vi "Leer.vi"(0 "VISA resource name out 2":refnum<visa-resource-name>, 1 "error out":errorcluster) -> (2 "Valor":dbl, 3 "VISA resource name out 3":refnum<visa-resource-name>, 4 "error out 2":errorcluster)   [LabVIEW 2015, in "Arduino GIERM.lvlib"]
uses:
  <instrlib>/Arduino GIERM/Arduino GIERM.lvlib
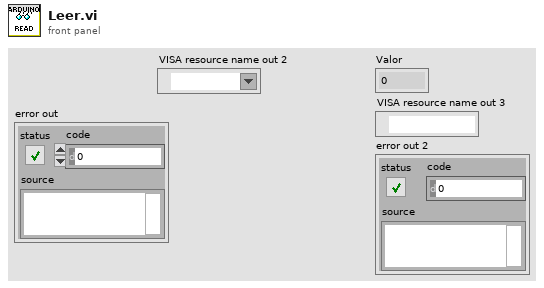
[diagram p1: front panel]
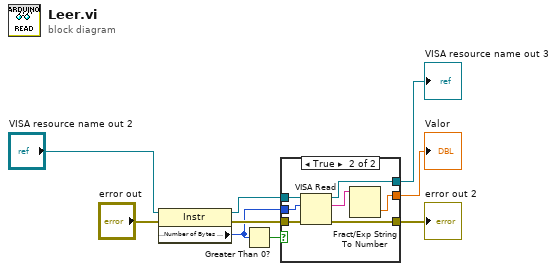
[diagram p0: block diagram]
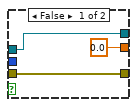
[diagram p2: hidden frame]
diagram:
  n1 = property class="Instr"(reference="VISA resource name out 2", error in="error out") -> (reference out=w5:refnum<visa-resource-name>, error out=w3:errorcluster, "Serial Settings:Number of Bytes at Serial Port"=w2:u32)
  n2 = Greater Than 0?(x=w2) -> (x > 0?=w1:bool)
  n3 = case shown="True" w1 {
    tunnel: w5 -> [w12 w19]
    tunnel: w3 -> [w11 w17]
    tunnel: [w12 w18] -> w8
    tunnel: [w11 w16] -> w7
    tunnel: w2 -> [_ w15]
    tunnel: [0.0 w13] -> w9
    frame False {
    }
    frame True {
      n4 = VISA Read(VISA resource name=w19, byte count=w15, error in (no error)=w17) -> (VISA resource name out=w18:refnum<visa-resource-name>, read buffer=w14:string, error out=w16:errorcluster)  [unwired: 1 out]
      n5 = Fract/Exp String To Number(string=w14) -> (number=w13:dbl)  [unwired: 3 in, 1 out]
    }
  }
  "Valor" <- w9
  "VISA resource name out 3" <- w8
  "error out 2" <- w7
